vi "Plot IV Response.vi"(8 "error in (no error)":errorcluster, 10 "Supply Line Handle in":refnum<k15>, 11 "Supply Line Measurements Results":T1) -> (0 "error out":errorcluster, 2 "Current Plot":waveform(dbl)(graph), 3 "Voltage Plot":waveform(dbl)(graph))   [LabVIEW 2018, in "RDLUtilities.lvlib"]
uses:
  RDLUtilities.lvlib
  Supply/Typedefs/Measurement Results.ctl
  Supply/Supply.lvlib
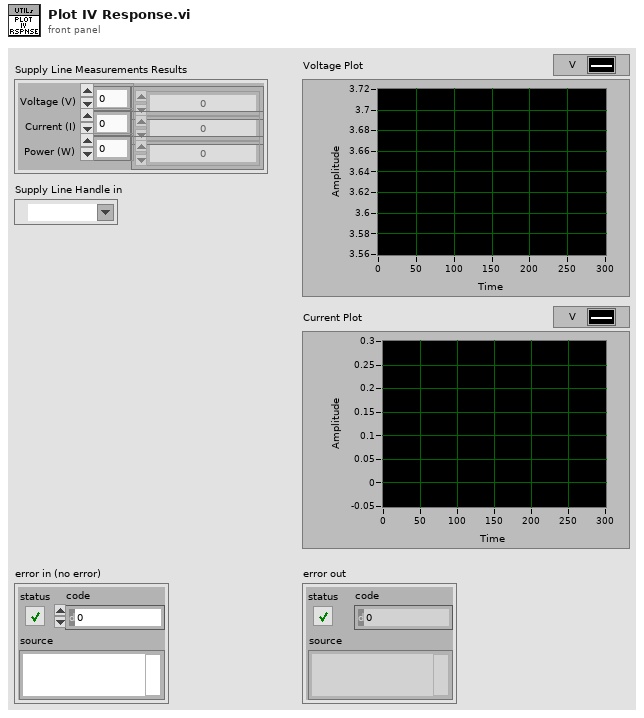
[diagram p1: front panel]
types:
  T1 = typedef "Supply.lvlib/Measurement Results.ctl" = cluster{"Voltage (V)":dbl[], "Current (I)":dbl[], "Power (W)":dbl[]}
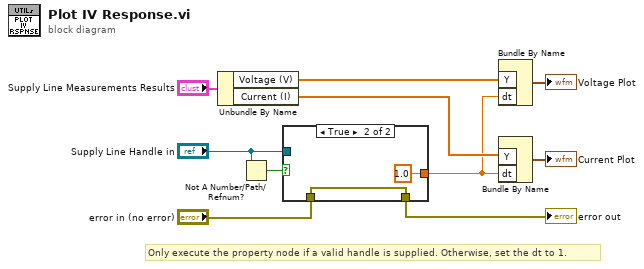
[diagram p0: block diagram]
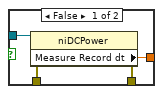
[diagram p2: hidden frame]
diagram:
  # "Only execute the property node if a valid handle is supplied. Otherwise, set the dt to 1."
  n1 = Unbundle By Name("Supply Line Measurements Results") -> ("Voltage (V)"=w7:dbl[], "Current (I)"=w6:dbl[])
  n2 = Not A Number/Path/Refnum?(number/path/refnum="Supply Line Handle in") -> (NaN/Path/Refnum?=w5:bool)
  n3 = case shown="True" w5 {
    tunnel: "error in (no error)" -> [w14 w16]
    tunnel: [w13 w16] -> w2
    tunnel: [w12 1.0 ("Measure Record dt")] -> w1
    tunnel: "Supply Line Handle in" -> [w11 _]
    frame False {
      n4 = property class="niDCPower"(reference=w11, error in=w14) -> (error out=w13:errorcluster, "Measure Record dt"=w12:dbl)  [unwired: 1 out]
    }
    frame True {
    }
  }
  "error out" <- w2
  n5 = Bundle By Name("Y"=w7, "dt"=w1) -> (→"Voltage Plot":waveform(dbl))  [unwired: 1 in]
  n6 = Bundle By Name("Y"=w6, "dt"=w1) -> (→"Current Plot":waveform(dbl))  [unwired: 1 in]
